vi "scan2d_initialize_detector.vi"(8 "error in (no error)":errorcluster, 11 "scan_2d in":refnum<class "scan_2d.lvclass">) -> (0 "error out":errorcluster, 3 "scan_2d out":refnum<class "scan_2d.lvclass">)   [LabVIEW 2015, in "scan_2d.lvclass"]
uses:
  scan_2d.lvclass
  UI/front_panel_class/hardware_caller_queue_numbers.ctl
  Detector_Class/detector/detector.lvclass
  scan_2d.lvclass/scan_2d.ctl
  UI/panel_class/panel.lvclass
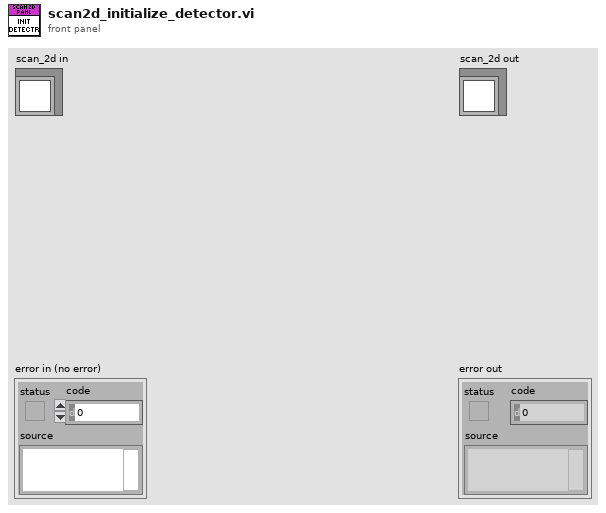
[diagram p1: front panel]
types:
  T1 = typedef "hardware_caller_queue_numbers.ctl" = enum16{"stage1", "stage2", "experiment", "detector"}
  T2 = typedef "data_types_tdef.ctl" = enum16{"0D", "1D", "2D"}
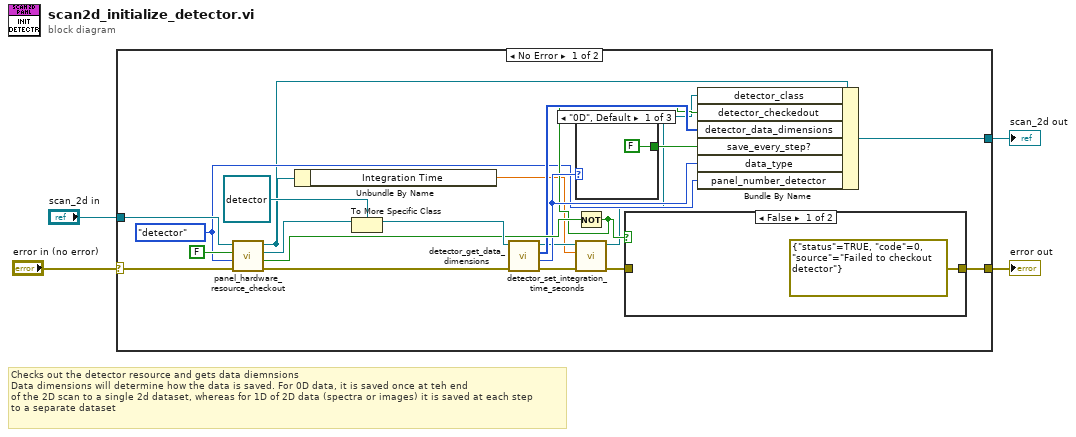
[diagram p0: block diagram]
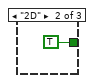
[diagram p3: hidden frame]
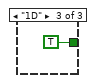
[diagram p4: hidden frame]
diagram:
  # "Checks out the detector resource and gets data diemnsions\nData dimensions will determine how the data is saved. For 0D data, it is saved once at teh end\nof the 2D scan to a single 2d dataset, whereas for 1D of 2D data (spectra or images) it is saved at each step\nto a separate dataset"
  n1 = case shown="No Error" "error in (no error)" {
    selector: "error in (no error)" -> [w23 w32]
    tunnel: [w12 w32] -> w3
    tunnel: [w18 w31] -> w1
    tunnel: "scan_2d in" -> [w21 w31]
    frame No Error {
      w11 = hardware_caller_queue_numbers."detector" ("panel_number")
      n2 = call "panel_hardware_resource_checkout.vi"("error in (no error)"=w23, "panel_number"=w11, "Self?"=FALSE, "panel in"=w21) -> ("error out"=w19:errorcluster, "timed out?"=w17:bool, "hardware.lvclass"=w22:refnum<class "hardware.lvclass">, "panel out"=w6:refnum<class "scan_2d.lvclass">)  [unwired: 4 in]
      n3 = Unbundle By Name(w6) -> ("Integration Time"=w5:dbl)
      n4 = To More Specific Class(target class=refnum<class "detector.lvclass"> refnum ("detector.lvclass"), reference=w22) -> (specific class reference=w20:refnum<class "detector.lvclass">)  [unwired: 1 in, 1 out]
      n5 = call-dynamic "detector_get_data_dimensions.vi"("error in (no error)"=w19, "detector in"=w20) -> ("error out"=w10:errorcluster, "data_type"=w14:T2, "dims"=w16:u32[], "detector out"=w8:refnum<class "detector.lvclass">)  [unwired: 6 in]
      n6 = case shown="\"0D\", Default" w14 {
        tunnel: [FALSE TRUE TRUE] -> w15
        frame "0D", Default {
        }
        frame "2D" {
        }
        frame "1D" {
        }
      }
      n7 = Not(x=w17) -> (.not. x?=w13:bool)
      n8 = call-dynamic "detector_set_integration_time_seconds.vi"("error in (no error)"=w10, "integration time (seconds)"=w5, "detector in"=w8) -> ("error out"=w9:errorcluster, "detector out"=w7:refnum<class "detector.lvclass">)  [unwired: 7 in]
      n9 = case shown="False" w13 {
        tunnel: w9 -> [_ w27]
        tunnel: [errorcluster {"status"=TRUE, "code"=0, "source"="Failed to checkout detector"} ("error out") w27] -> w12
        frame False {
        }
        frame True {
        }
      }
      n10 = Bundle By Name(cluster=w6, "detector_class"=w7, "detector_checkedout"=w13, "detector_data_dimensions"=w16, "save_every_step?"=w15, "data_type"=w14, "panel_number_detector"=w11) -> (w18:refnum<class "scan_2d.lvclass">)
    }
    frame Error {
    }
  }
  "error out" <- w3
  "scan_2d out" <- w1
